vi "splitAndSum.vi"(11 "Real Matrix":T1) -> (1 "Array":dbl[][](array[numeric]), 2 "columns":i32, 3 "rows":i32)   [LabVIEW 2015]
uses:
  <vilib>/Analysis/Matrix/Datatypes/RealMatrix.ctl
  <vilib>/Analysis/Matrix/Numeric/Conversions/Matrix To Array - RM.vi
  <vilib>/Analysis/Matrix/NI_Matrix.lvlib
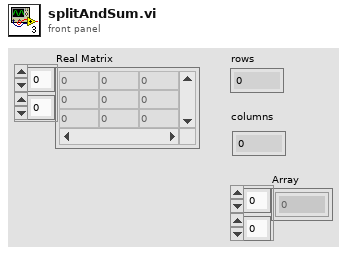
[diagram p1: front panel]
types:
  T1 = typedef "NI_Matrix.lvlib/RealMatrix.ctl" = dbl[][]
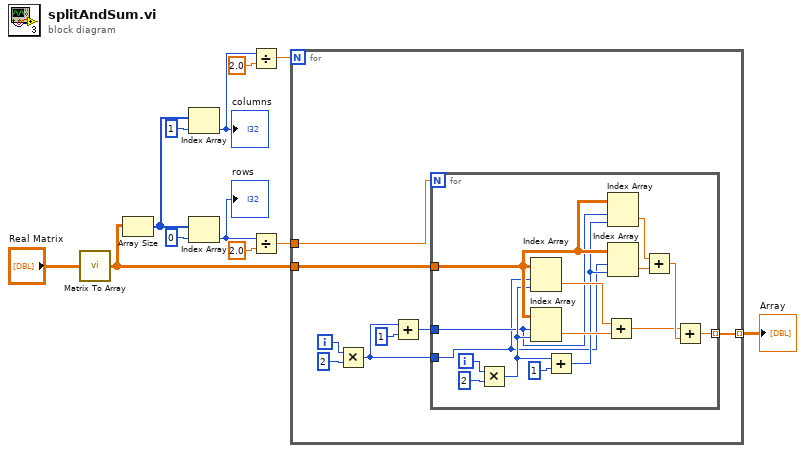
[diagram p0: block diagram]
diagram:
  n1 = call-poly <vilib>:"Matrix To Array.vi"("Real Matrix"="Real Matrix") -> ("Real 2D Array"=w5:dbl[][])
  n2 = Array Size(array=w5) -> (size(s)=w3:i32[])
  n3 = Index Array(array=w3, index=1) -> (element=w12:i32)
  "columns" <- w12
  n4 = Index Array(array=w3, index=0) -> (element=w11:i32)
  "rows" <- w11
  n5 = Divide(x=w12, y=2.0) -> (x/y=w7:dbl)
  n6 = Divide(x=w11, y=2.0) -> (x/y=w8:dbl)
  n7 = for {
    N: w7 -> [_]
    tunnel: w5 -> [w20]
    tunnel: w8 -> [w17]
    tunnel: [w13] -> w6 mode=indexing
    i -> [w19]
    n8 = Multiply(x=w19, y=2) -> (x*y=w16:i32)
    n9 = Add(x=w16, y=1) -> (x+y=w14:i32)
    n10 = for {
      N: w17 -> [_]
      tunnel: w16 -> [w21]
      tunnel: w20 -> [w32]
      tunnel: w14 -> [w23]
      tunnel: [w25] -> w13 mode=indexing
      i -> [w34]
      n11 = Multiply(x=w34, y=2) -> (x*y=w24:i32)
      n12 = Index Array(array=w32, index (row)=w21, index (col)=w24) -> (element=w31:dbl)
      n13 = Index Array(array=w32, index (row)=w23, index (col)=w24) -> (element=w30:dbl)
      n14 = Add(x=w24, y=1) -> (x+y=w22:i32)
      n15 = Add(x=w31, y=w30) -> (x+y=w26:dbl)
      n16 = Index Array(array=w32, index (row)=w23, index (col)=w22) -> (element=w28:dbl)
      n17 = Index Array(array=w32, index (row)=w21, index (col)=w22) -> (element=w29:dbl)
      n18 = Add(x=w28, y=w29) -> (x+y=w27:dbl)
      n19 = Add(x=w26, y=w27) -> (x+y=w25:dbl)
    }
  }
  "Array" <- w6
